vi "Read Firmware Valid.vi"(8 "error in (no error)":errorcluster, 11 "DCM - RT in":refnum<class "DCM - RT.lvclass">) -> (0 "error out":errorcluster, 2 "Firmware Valid":bool, 3 "DCM - RT out":refnum<class "DCM - RT.lvclass">)   [LabVIEW 2016, in "DCM-Classes.lvlib" / "DCM - RT.lvclass"]
uses:
  DCM - RT.lvclass
  DCM - RT.lvclass/DCM - RT.ctl
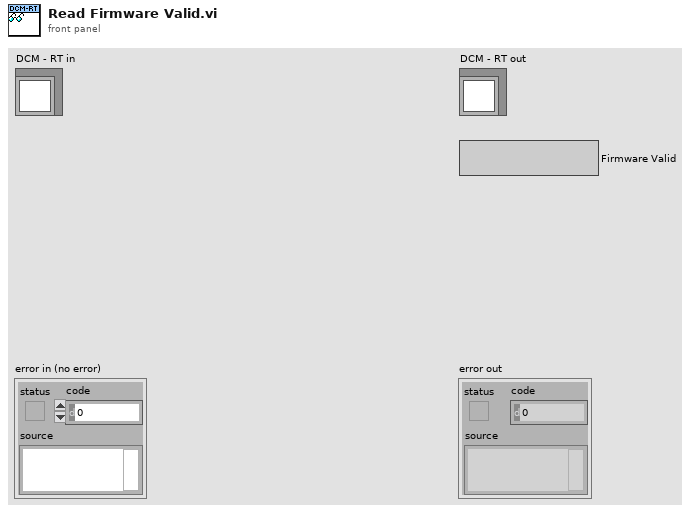
[diagram p1: front panel]
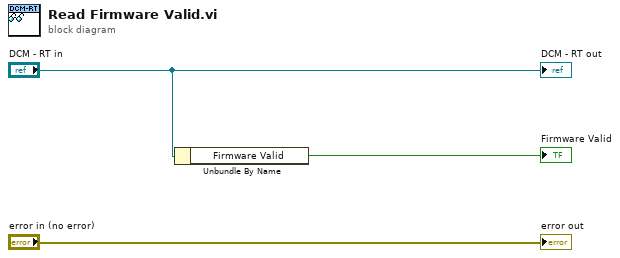
[diagram p0: block diagram]
diagram:
  n1 = Unbundle By Name("DCM - RT in") -> ("Firmware Valid"=→"Firmware Valid":bool)
  "error out" <- "error in (no error)"
  "DCM - RT out" <- "DCM - RT in"
